vi "Blank.vi"() -> ()   [LabVIEW 2020]
uses:
  <vilib>/DAQmx/read.llb/DAQmx Read (Analog 2D DBL NChan NSamp).vi
  <vilib>/DAQmx/miscellaneous.llb/DAQmx Fill In Error Info.vi
panel:
  in  "Read Time (s)":i32
  in  "stop 3":bool
  out "Array 2":dbl[][](array[numeric])
  in  "stop 2":bool
  in  "Sampling Time (s)":dbl=1.0 caption="Delay Time (s)"
  out "Array":dbl[][](array[numeric])
  in  "DAQmx Task Name":refnum<k21>
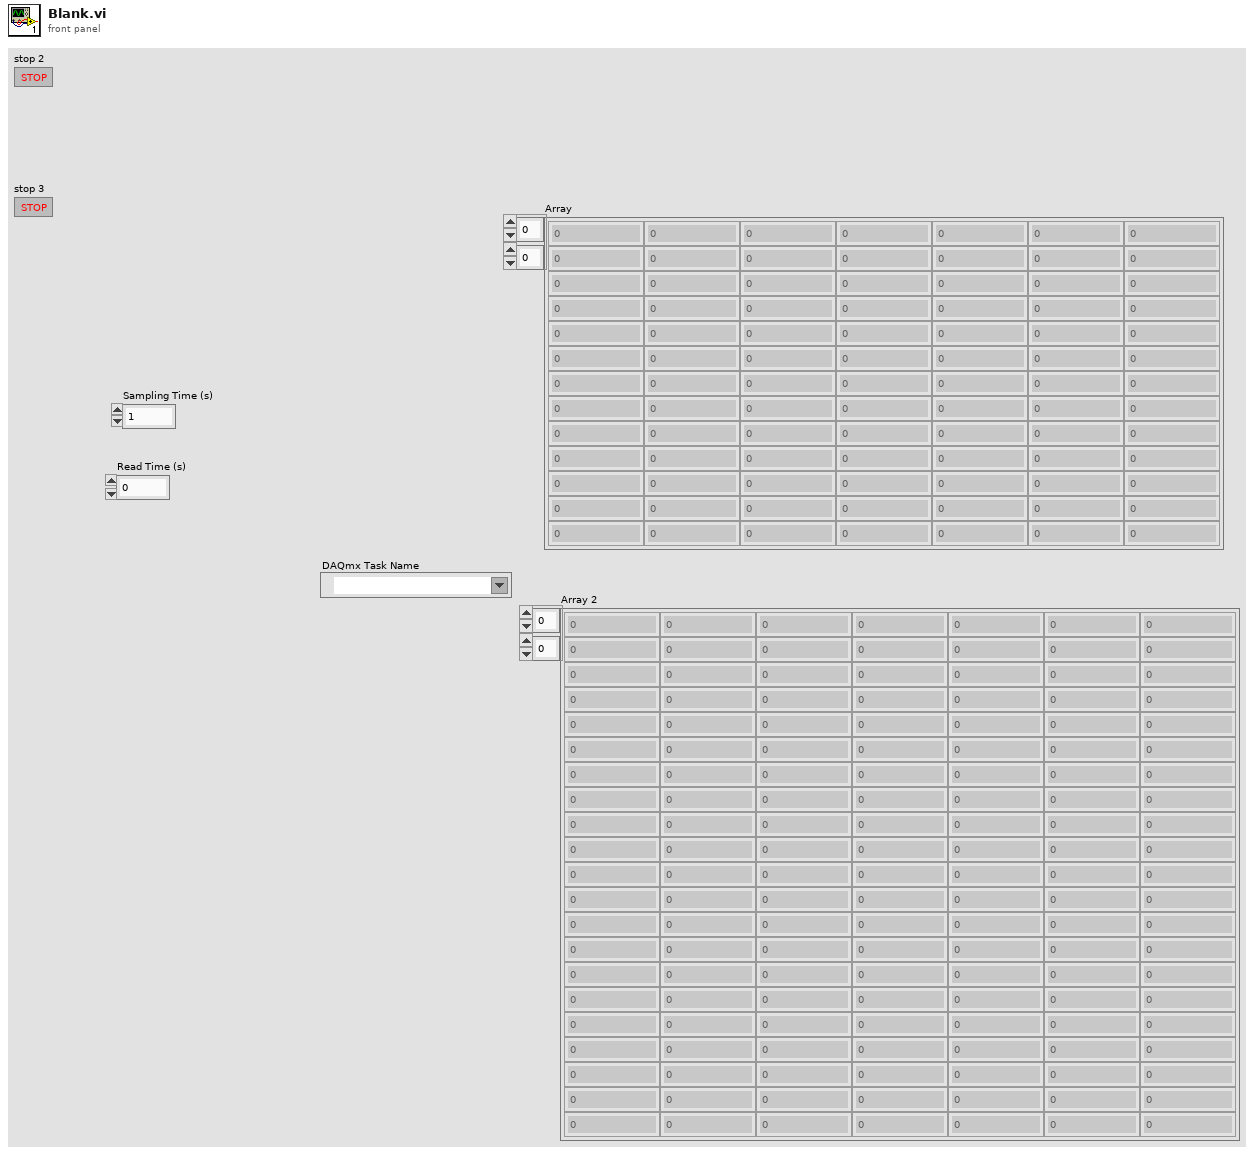
[diagram p1: front panel]
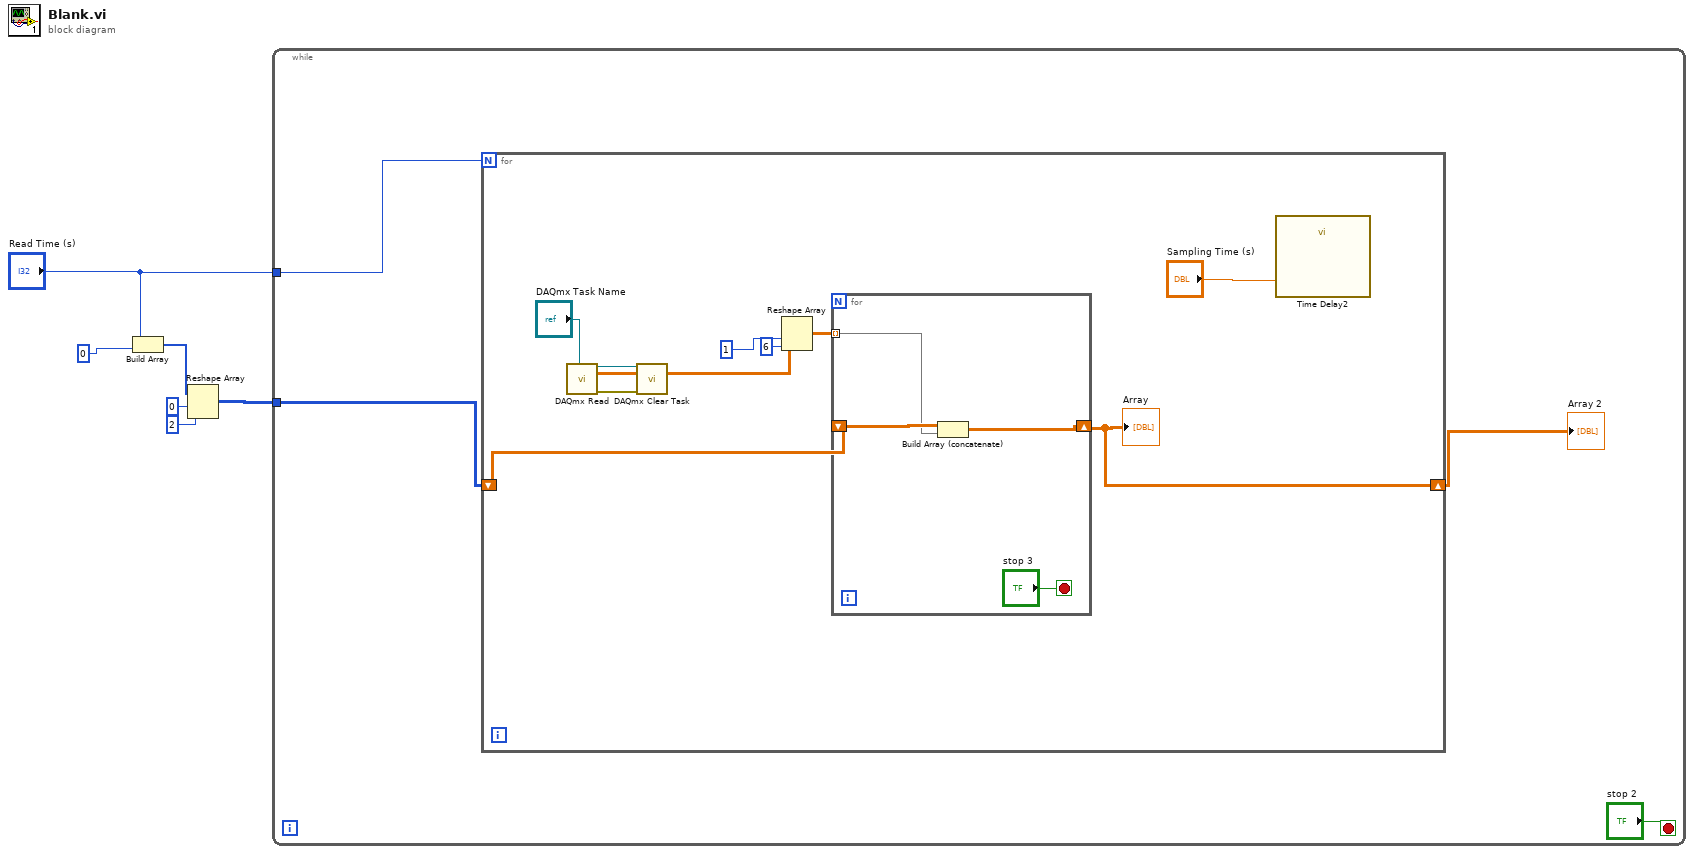
[diagram p0: block diagram]
diagram:
  n1 = Build Array("Read Time (s)", 0 ("element")) -> (w5:i32[])
  n2 = Reshape Array(w5, 0 ("dimension size"), 2 ("dimension size")) -> (w2:i32[][])
  n3 = while {
    tunnel: "Read Time (s)" -> [w8]
    tunnel: w2 -> [w7]
    stop <- "stop 2" stop-if-true
    n4 = for {
      N: w8 -> [_]
      shift-right: [w12] -> w9
      shift-left: w7 -> [w11]
      n5 = call-poly <vilib>:"DAQmx Read.vi"("task/channels in"="DAQmx Task Name") -> ("task out"=w19:refnum<k21>, "data"=w14:dbl[][], "error out"=w20:errorcluster)  [unwired: 12 in]
      n6 = call <vilib>:"DAQmx Clear Task.vi"("task in"=w19, "error in"=w20) -> ()  [unwired: 13 in, 1 out]
      n7 = Reshape Array(w14, 1 ("dimension size"), 6 ("dimension size")) -> (w13:dbl[][])
      n8 = for {
        shift-right: [w23] -> w12
        shift-left: w11 -> [w24]
        tunnel: w13 -> [w22] mode=indexing
        stop <- "stop 3" stop-if-true
        n9 = Build Array (concatenate)(w24, w22) -> (w23:dbl[][])
      }
      "Array" <- w12
      n10 = call "Time Delay2"("Delay Time (s)"="Sampling Time (s)") -> ()  [unwired: 10 in, 1 out]
    }
    "Array 2" <- w9
  }
